vi "Write Display Format.vi"(8 "error in (no error)":errorcluster, 10 "DisplayFormat":T1, 11 "Digital.lvclass in":refnum<class "Digital.lvclass">) -> (0 "error out":errorcluster, 3 "Digital.lvclass out":refnum<class "Digital.lvclass">)   [LabVIEW 2015, in "Digital.lvclass"]
uses:
  Digital.lvclass
  <vilib>/Utility/miscctls.llb/LVFormatAndPrecisionTypeDef.ctl
  Digital.lvclass/Digital.ctl
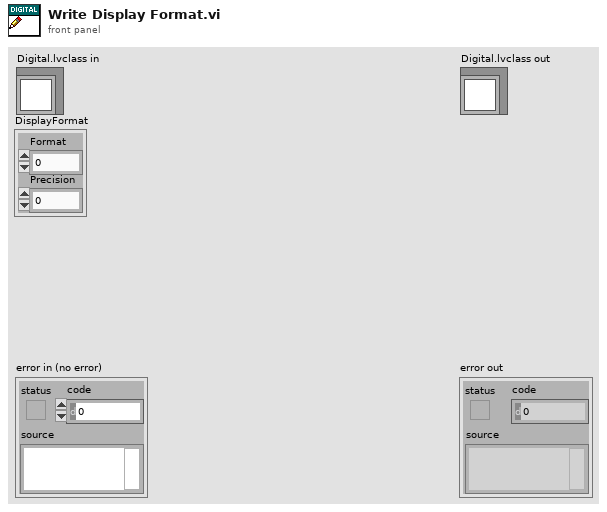
[diagram p1: front panel]
types:
  T1 = typedef "LVFormatAndPrecisionTypeDef.ctl" = cluster{"Format":u8, "Precision":u8}
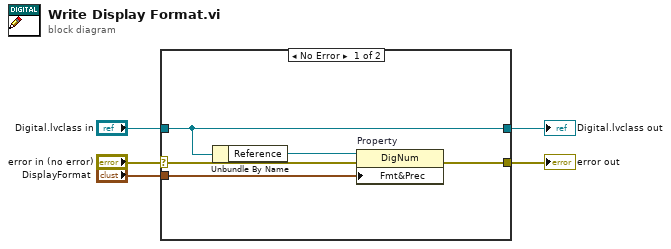
[diagram p0: block diagram]
diagram:
  n1 = case shown="No Error" "error in (no error)" {
    selector: "error in (no error)" -> [w6 w12]
    tunnel: [w10 w12] -> w4
    tunnel: [w8 w11] -> w2
    tunnel: "Digital.lvclass in" -> [w8 w11]
    tunnel: "DisplayFormat" -> [w9 _]
    frame No Error {
      n2 = Unbundle By Name(w8) -> ("Reference"=w7:refnum<vi>)
      n3 = property on="Property" class="DigNum"(reference=w7, error in=w6, "Fmt&Prec"=w9) -> (error out=w10:errorcluster)  [unwired: 1 out]
    }
    frame Error {
    }
  }
  "error out" <- w4
  "Digital.lvclass out" <- w2
